vi "Feeder_Determiner.vi"() -> ()   [LabVIEW 2020]
uses:
  <vilib>/Rock Robotics/WPI/DriverStation/WPI_DriverStationRobotMode2.ctl
  Feeder_Control_States.ctl
  Subsystems/Funnel/Funnel_Cluster.ctl
  Subsystems/Funnel/Control_States_Funnel.ctl
  Subsystems/Magazine/Magazine_Cluster.ctl
  Subsystems/Magazine/Magazine_Control_States.ctl
  Subsystems/Intake/Intake_cluster.ctl
  Subsystems/Intake/Intake_control_states.ctl
  Globals/Feeder_Globals.vi
  Globals/Funnel_global.vi
  Globals/Magazine_Globals.vi
  Globals/Intake_Globals.vi
  Robot Global Data.vi
  Globals/Sensor_Values.vi
  Globals/Flywheel_Globals.vi
  Globals/Cowl_Globals.vi
  Shooter/Determiner/Shooter_Globals.vi
  Globals/Turret_Globals.vi
panel:
  in  "Intake_Outtake_%Vbus":dbl=-0.5
  in  "Magazine_Outtake_%Vbus":dbl=-0.3
  in  "Funnel_Outtake_%Vbus":dbl=-0.5
  in  "use magazine speed control test":bool
  in  "Magazine_Speed_Control_Test_Value":dbl=6000.0
  in  "Intake_Load_%Vbus":dbl=0.5
  in  "Magazine_Load_%Vbus":dbl=0.3
  in  "Funnel_Load_%Vbus":dbl=0.7
  in  "Funnel_Firing_%Vbus":dbl=0.5
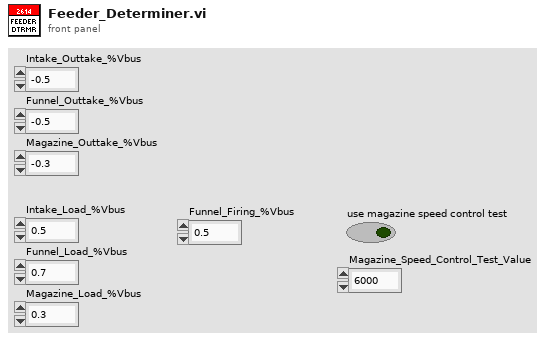
[diagram p1: front panel]
types:
  T1 = typedef "Feeder_Control_States.ctl" = enum16{"No-Op", "Manual", "Load", "Outtake", "Firing", "Test", "Command_Feed", "Command_Shoot", "Puke-Op", "Command_Feed_From_Pose", "Load+Firing", "Command_Puke"}
  T2 = typedef "Intake_cluster.ctl" = cluster{"control_states":T3, "%Vbus":dbl, "Trigger?":bool, "Manual_Extend?":bool, "Auto_Notifier":refnum<notifier>, "Step":dbl, "Parameter 1":dbl, "Parameter 2":dbl, "Parameter 3":dbl}
  T3 = typedef "Intake_control_states.ctl" = enum16{"No_Op", "Intake", "Manual", "Outtake", "Extend_No_Motor", "Retract_No_Motor"}
  T4 = typedef "Magazine_Cluster.ctl" = cluster{"Control_States":T5, "%Vbus":dbl, "Load_Magazine":bool, "Firing_Magazine":bool, "Velocity":dbl}
  T5 = typedef "Magazine_Control_States.ctl" = enum16{"No-Op", "Manual_%Vbus", "Manual_Speed_Control", "Test_Speed_Control", "Load", "Firing", "Outtake"}
  T6 = typedef "Funnel_Cluster.ctl" = cluster{"Control States":T7, "%Vbus":dbl}
  T7 = typedef "Control_States_Funnel.ctl" = enum16{"No_Op", "Manual_Op", "Load", "Firing", "Outtake"}
  T8 = typedef "WPI_DriverStationRobotMode2.ctl" = enum16{"Autonomous Disabled", "Autonomous Enabled", "Teleop Disabled", "Teleop Enabled", "Disconnected", "Finish", "Test Disabled", "Test Enabled", "Emergency Stopped"}
  T9 = typedef "Feeder_Cluster.ctl" = cluster{"Firing":bool, "Load":bool, "Magazine_%Vbus":dbl, "Funnel_%Vbus":dbl, "Intake_%Vbus":dbl, "Manual_Extend":bool, "Outtake":bool, "Parameters":dbl[], "Auto_Notifier":refnum<notifier>, "Step":i32, "Control_States":T1, "Puke?":bool}
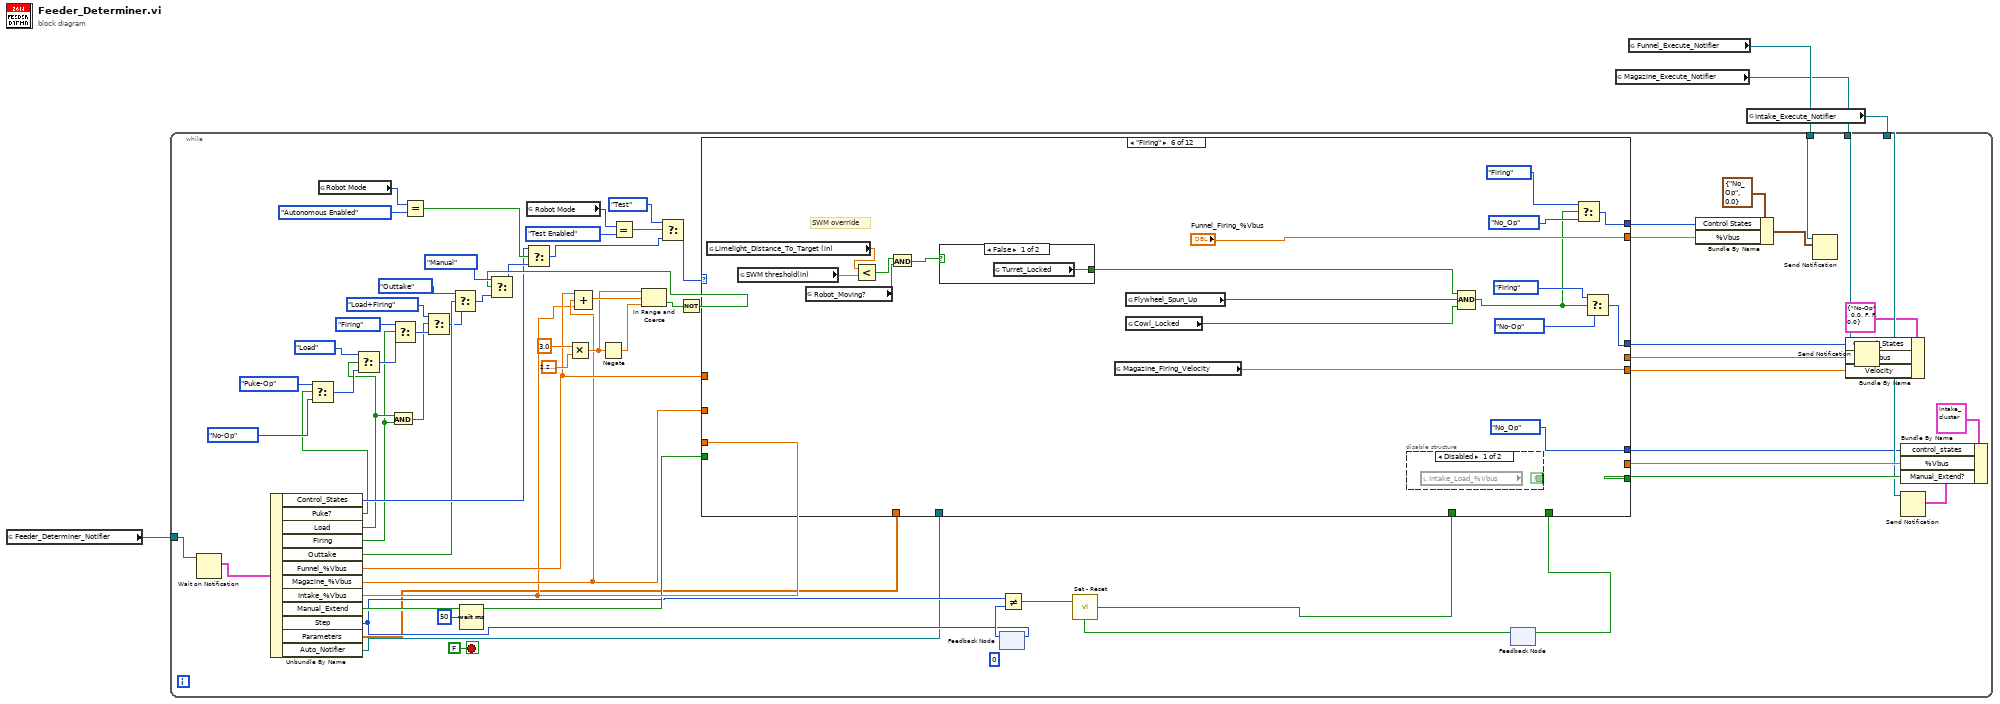
[diagram p0: block diagram]
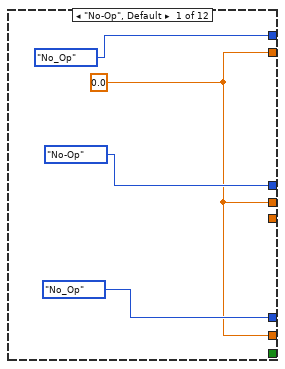
[diagram p2: hidden frame]
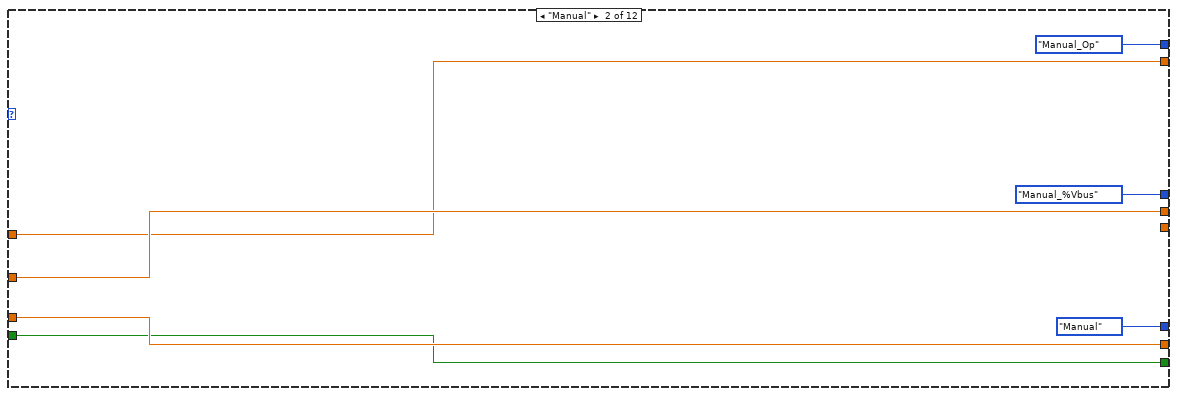
[diagram p3: hidden frame]
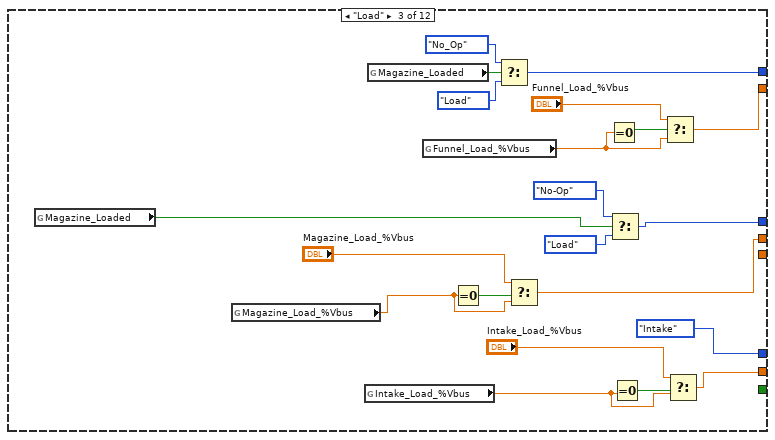
[diagram p4: hidden frame]
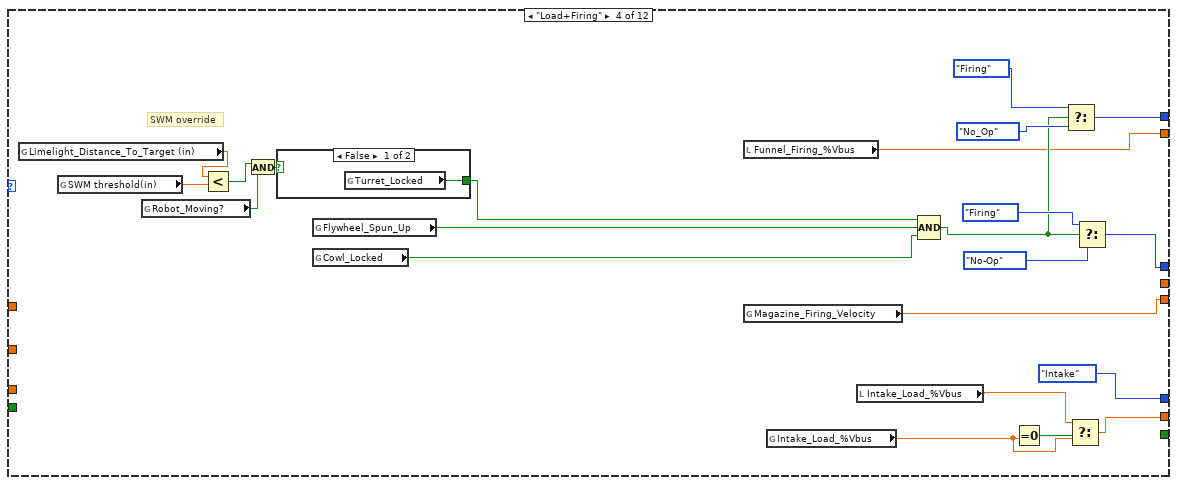
[diagram p5: hidden frame]
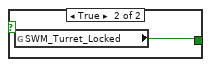
[diagram p6: hidden frame]
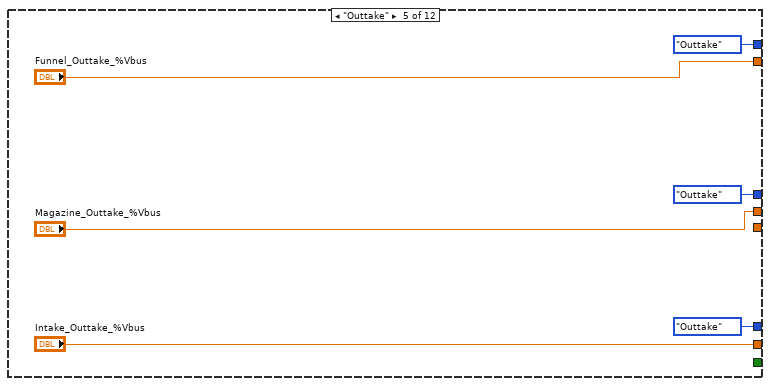
[diagram p7: hidden frame]
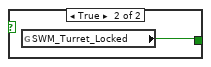
[diagram p8: hidden frame]
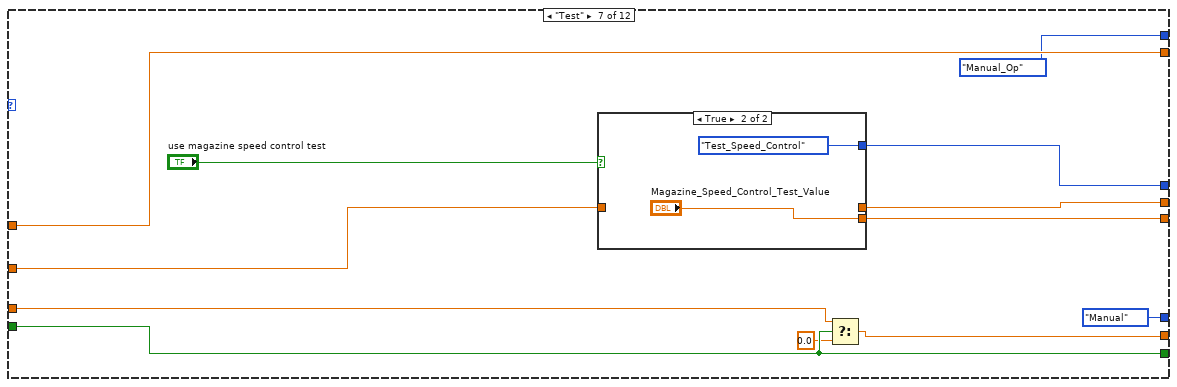
[diagram p10: hidden frame]
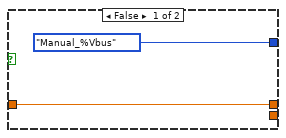
[diagram p11: hidden frame]
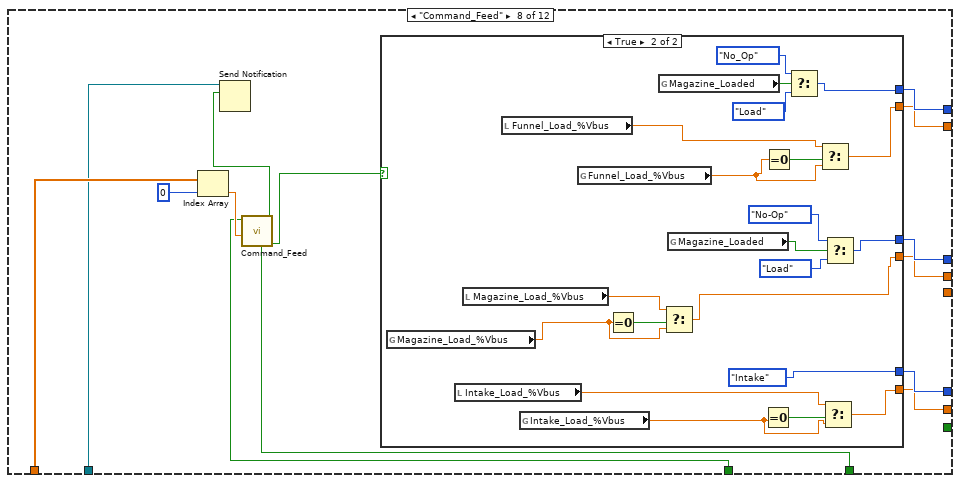
[diagram p12: hidden frame]
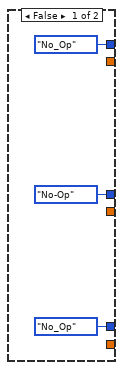
[diagram p13: hidden frame]
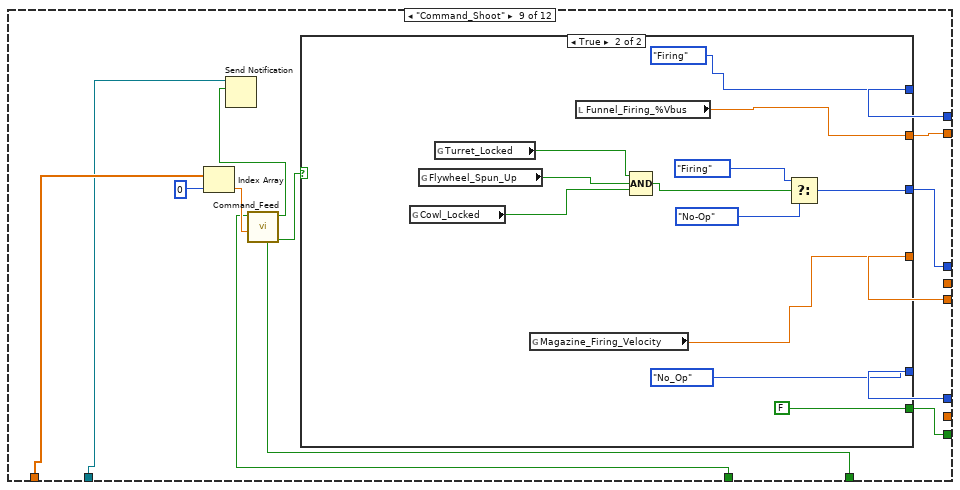
[diagram p14: hidden frame]
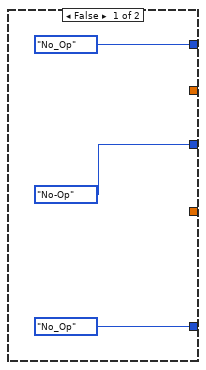
[diagram p15: hidden frame]
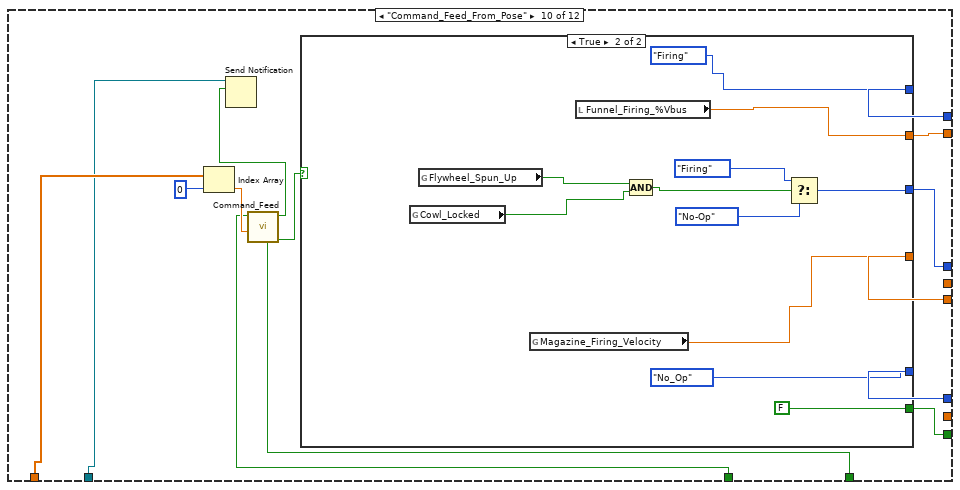
[diagram p16: hidden frame]
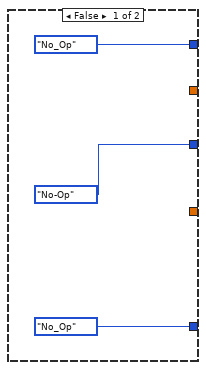
[diagram p17: hidden frame]
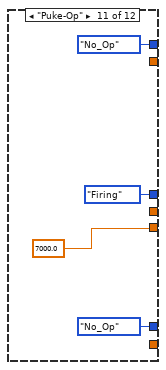
[diagram p18: hidden frame]
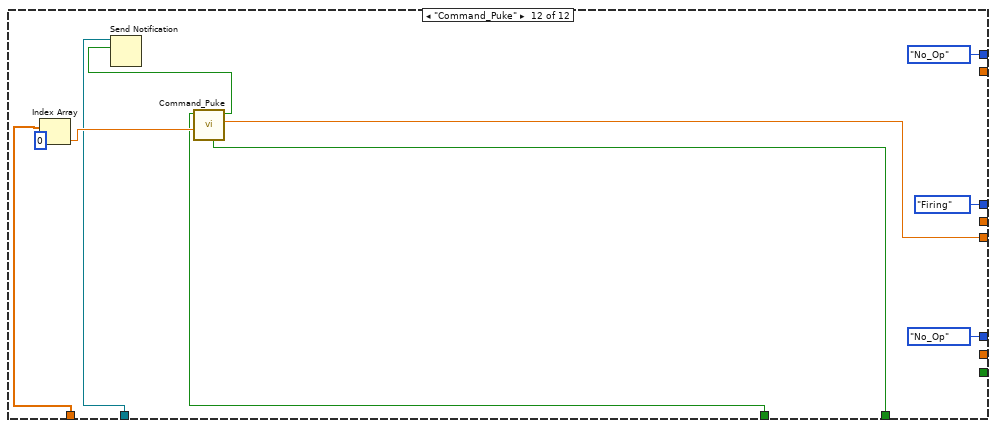
[diagram p19: hidden frame]
diagram:
  n1 = global read "Feeder_Globals.vi" "Feeder_Determiner_Notifier"() -> (w4:refnum<notifier>)
  n2 = global read "Magazine_Globals.vi" "Magazine_Execute_Notifier"() -> (w2:refnum<notifier>)
  n3 = global read "Funnel_global.vi" "Funnel_Execute_Notifier"() -> (w3:refnum<notifier>)
  n4 = global read "Intake_Globals.vi" "Intake_Execute_Notifier"() -> (w1:refnum<notifier>)
  n5 = while {
    tunnel: w4 -> [w71]
    tunnel: w3 -> [w59]
    tunnel: w2 -> [w58]
    tunnel: w1 -> [w57]
    stop <- FALSE stop-if-true
    (unwired) 0 ("Step")
    n6 = Wait on Notification(notifier=w71) -> (notification=w15:T9)  [unwired: 3 in, 3 out]
    n7 = Unbundle By Name(w15) -> ("Control_States"=w24:T1, "Puke?"=w9:bool, "Load"=w11:bool, "Firing"=w10:bool, "Outtake"=w23:bool, "Funnel_%Vbus"=w22:dbl, "Magazine_%Vbus"=w21:dbl, "Intake_%Vbus"=w20:dbl, "Manual_Extend"=w19:bool, "Step"=w18:i32, "Parameters"=w17:dbl[], "Auto_Notifier"=w16:refnum<notifier>)
    n8 = Select(t=Feeder_Control_States."Puke-Op", s=w9, f=Feeder_Control_States."No-Op" ("Control_States")) -> (s? t:f=w14:T1)
    n9 = global read "Robot Global Data.vi" "Robot Mode"() -> (w46:T8)
    n10 = Select(t=Feeder_Control_States."Load" ("Control_States"), s=w11, f=w14) -> (s? t:f=w67:T1)
    n11 = And(x=w11, y=w10) -> (x .and. y?=w7:bool)
    n12 = Select(t=Feeder_Control_States."Firing" ("Control_States"), s=w10, f=w67) -> (s? t:f=w8:T1)
    n13 = Equal?(x=w46, y=WPI_DriverStationRobotMode2."Autonomous Enabled" ("Robot Mode")) -> (x = y?=w35:bool)
    n14 = Select(t=Feeder_Control_States."Load+Firing" ("Control_States"), s=w7, f=w8) -> (s? t:f=w5:T1)
    n15 = Select(t=Feeder_Control_States."Outtake" ("Control_States"), s=w23, f=w5) -> (s? t:f=w34:T1)
    n16 = Wait (ms)(milliseconds to wait=u32 50) -> ()  [unwired: 1 out]
    n17 = global read "Robot Global Data.vi" "Robot Mode"() -> (w69:T8)
    n18 = Multiply(x=3.0, y=2.220446049250313e-16) -> (x*y=w28:dbl)
    n19 = Compound Arithmetic op=ADD(w22, w21, w20) -> (w32:dbl)
    n20 = Negate(x=w28) -> (-x=w31:dbl)
    n21 = Equal?(x=w69, y=WPI_DriverStationRobotMode2."Test Enabled" ("Robot Mode")) -> (x = y?=w68:bool)
    n22 = In Range and Coerce(upper limit=w28, x=w32, lower limit=w31) -> (In Range?=w27:bool)  [unwired: 1 out]
    n23 = Not(x=w27) -> (.not. x?=w26:bool)
    n24 = Select(t=Feeder_Control_States."Manual", s=w26, f=w34) -> (s? t:f=w25:T1)
    n25 = Select(t=w24, s=w35, f=w25) -> (s? t:f=w45:T1)
    n26 = Select(t=Feeder_Control_States."Test" ("Control_States"), s=w68, f=w45) -> (s? t:f=w60:T1)
    n27 = feedback #1() -> (w42:i32)  [unwired: 1 in]
    n28 = feedback-in #1(w18) -> ()
    n29 = Not Equal?(x=w18, y=w42) -> (x != y?=w43:bool)
    n30 = feedback #2() -> (w44:bool)  [unwired: 1 in]
    n31 = call "Set - Reset.vi"("Reset"=w44, "Set"=w43) -> ("Output"=w40:bool)
    n32 = case shown="\"Firing\"" w60 {
      tunnel: [Magazine_Control_States."No-Op" ("Control_States") Magazine_Control_States."Manual_%Vbus" ("Control_States") w97 w112 Magazine_Control_States."Outtake" ("Control_States") w149 w167 w176 w214 w243 Magazine_Control_States."Firing" ("Control_States") Magazine_Control_States."Firing" ("Control_States")] -> w64
      tunnel: [Intake_control_states."No_Op" ("control_states") Intake_control_states."Manual" ("control_states") Intake_control_states."Intake" ("control_states") Intake_control_states."Intake" ("control_states") Intake_control_states."Outtake" ("control_states") Intake_control_states."No_Op" ("control_states") Intake_control_states."Manual" ("control_states") w175 w211 w240 Intake_control_states."No_Op" ("control_states") Intake_control_states."No_Op" ("control_states")] -> w37
      tunnel: [w74 w82 w84 w123 "Intake_Outtake_%Vbus" _ w157 w172 _ _ _ _] -> w62
      tunnel: [_ w81 _ _ _ _ w159 _ w215 w244 _ _] -> w61
      tunnel: w22 -> [_ w79 _ _ _ _ w166 _ _ _ _ _]
      tunnel: [w74 w79 w92 w114 "Funnel_Outtake_%Vbus" "Funnel_Firing_%Vbus" w166 w174 w210 w239 _ _] -> w56
      tunnel: w21 -> [_ w83 _ _ _ _ w165 _ _ _ _ _]
      tunnel: [w74 w83 w88 _ "Magazine_Outtake_%Vbus" _ w163 w173 _ _ _ _] -> w55
      tunnel: w20 -> [_ w82 _ _ _ _ w158 _ _ _ _ _]
      tunnel: w19 -> [_ w81 _ _ _ _ w159 _ _ _ _ _]
      tunnel: [_ _ _ w111 _ w141 w162 _ w213 w242 7000.0 ("Magazine_Firing_Velocity") w271] -> w53
      tunnel: [Control_States_Funnel."No_Op" ("Control States") Control_States_Funnel."Manual_Op" ("Control States") w96 w113 Control_States_Funnel."Outtake" ("Control States") w145 Control_States_Funnel."Manual_Op" ("Control States") w177 w212 w241 Control_States_Funnel."No_Op" ("Control States") Control_States_Funnel."No_Op" ("Control States")] -> w48
      tunnel: w17 -> [_ _ _ _ _ _ _ w185 w219 w248 _ w280]
      tunnel: w40 -> [_ _ _ _ _ _ _ w182 w216 w245 _ w278]
      tunnel: [_ _ _ _ _ _ _ w181 w217 w246 _ w277] -> w41
      tunnel: w16 -> [_ _ _ _ _ _ _ w180 w218 w247 _ w275]
      frame "No-Op", Default {
        w74 = 0.0 ("Throttle")
      }
      frame "Manual" {
      }
      frame "Load" {
        n33 = global read "Sensor_Values.vi" "Magazine_Loaded"() -> (w100:bool)
        n34 = global read "Feeder_Globals.vi" "Magazine_Load_%Vbus"() -> (w89:dbl)
        n35 = global read "Feeder_Globals.vi" "Intake_Load_%Vbus"() -> (w85:dbl)
        n36 = global read "Sensor_Values.vi" "Magazine_Loaded"() -> (w101:bool)
        n37 = global read "Feeder_Globals.vi" "Funnel_Load_%Vbus"() -> (w93:dbl)
        n38 = Equal To 0?(x=w89) -> (x = 0?=w90:bool)
        n39 = Select(t=Control_States_Funnel."No_Op" ("Control States"), s=w101, f=Control_States_Funnel."Load" ("Control States")) -> (s? t:f=w96:T7)
        n40 = Select(t="Magazine_Load_%Vbus", s=w90, f=w89) -> (s? t:f=w88:dbl)
        n41 = Equal To 0?(x=w93) -> (x = 0?=w95:bool)
        n42 = Select(t=Magazine_Control_States."No-Op" ("Control_States"), s=w100, f=Magazine_Control_States."Load" ("Control_States")) -> (s? t:f=w97:T5)
        n43 = Equal To 0?(x=w85) -> (x = 0?=w87:bool)
        n44 = Select(t="Funnel_Load_%Vbus", s=w95, f=w93) -> (s? t:f=w92:dbl)
        n45 = Select(t="Intake_Load_%Vbus", s=w87, f=w85) -> (s? t:f=w84:dbl)
      }
      frame "Load+Firing" {
        # "SWM override"
        n46 = global read "Sensor_Values.vi" "Limelight_Distance_To_Target (in)"() -> (w108:dbl)
        n47 = global read "Shooter_Globals.vi" "SWM threshold(in)"() -> (w107:dbl)
        n48 = global read "Sensor_Values.vi" "Robot_Moving?"() -> (w109:bool)
        n49 = Less?(x=w108, y=w107) -> (x < y?=w106:bool)
        n50 = And(x=w106, y=w109) -> (x .and. y?=w110:bool)
        n51 = case shown="False" w110 {
          tunnel: [w127 w128] -> w105
          frame False {
            n52 = global read "Turret_Globals.vi" "Turret_Locked"() -> (w127:bool)
          }
          frame True {
            n53 = global read "Turret_Globals.vi" "SWM_Turret_Locked"() -> (w128:bool)
          }
        }
        n54 = global read "Flywheel_Globals.vi" "Flywheel_Spun_Up"() -> (w117:bool)
        n55 = global read "Cowl_Globals.vi" "Cowl_Locked"() -> (w115:bool)
        n56 = local read "Funnel_Firing_%Vbus"() -> (w114:dbl)
        n57 = global read "Feeder_Globals.vi" "Magazine_Firing_Velocity"() -> (w111:dbl)
        n58 = global read "Feeder_Globals.vi" "Intake_Load_%Vbus"() -> (w124:dbl)
        n59 = local read "Intake_Load_%Vbus"() -> (w122:dbl)
        n60 = Compound Arithmetic op=AND(w105, w117, w115) -> (w116:bool)
        n61 = Equal To 0?(x=w124) -> (x = 0?=w125:bool)
        n62 = Select(t=Control_States_Funnel."Firing" ("Control States"), s=w116, f=Control_States_Funnel."No_Op" ("Control States")) -> (s? t:f=w113:T7)
        n63 = Select(t=w122, s=w125, f=w124) -> (s? t:f=w123:dbl)
        n64 = Select(t=Magazine_Control_States."Firing" ("Control_States"), s=w116, f=Magazine_Control_States."No-Op" ("Control_States")) -> (s? t:f=w112:T5)
      }
      frame "Outtake" {
      }
      frame "Firing" {
        # "SWM override"
        n65 = global read "Sensor_Values.vi" "Limelight_Distance_To_Target (in)"() -> (w137:dbl)
        n66 = global read "Shooter_Globals.vi" "SWM threshold(in)"() -> (w136:dbl)
        n67 = global read "Sensor_Values.vi" "Robot_Moving?"() -> (w138:bool)
        n68 = Less?(x=w137, y=w136) -> (x < y?=w135:bool)
        n69 = And(x=w135, y=w138) -> (x .and. y?=w139:bool)
        n70 = case shown="False" w139 {
          tunnel: [w153 w154] -> w140
          frame False {
            n71 = global read "Turret_Globals.vi" "Turret_Locked"() -> (w153:bool)
          }
          frame True {
            n72 = global read "Turret_Globals.vi" "SWM_Turret_Locked"() -> (w154:bool)
          }
        }
        n73 = global read "Feeder_Globals.vi" "Magazine_Firing_Velocity"() -> (w141:dbl)
        n74 = global read "Flywheel_Globals.vi" "Flywheel_Spun_Up"() -> (w144:bool)
        n75 = global read "Cowl_Globals.vi" "Cowl_Locked"() -> (w142:bool)
        n76 = disable-structure shown="Disabled" {
          disable-tunnel: [FALSE ("intake_extended") _] -> _
          frame Disabled {
            n77 = local read "Intake_Load_%Vbus"() -> ()  [unwired: 1 out]
          }
          frame Enabled {
          }
        }
        n78 = Compound Arithmetic op=AND(w140, w144, w142) -> (w143:bool)
        n79 = Select(t=Control_States_Funnel."Firing" ("Control States"), s=w143, f=Control_States_Funnel."No_Op" ("Control States")) -> (s? t:f=w145:T7)
        n80 = Select(t=Magazine_Control_States."Firing" ("Control_States"), s=w143, f=Magazine_Control_States."No-Op" ("Control_States")) -> (s? t:f=w149:T5)
      }
      frame "Test" {
        n81 = case shown="True" "use magazine speed control test" {
          tunnel: [Magazine_Control_States."Manual_%Vbus" ("Control_States") Magazine_Control_States."Test_Speed_Control" ("Control_States")] -> w167
          tunnel: [w168 _] -> w163
          tunnel: w165 -> [w168 _]
          tunnel: [_ "Magazine_Speed_Control_Test_Value"] -> w162
          frame False {
          }
          frame True {
          }
        }
        n82 = Select(t=w158, s=w159, f=0.0) -> (s? t:f=w157:dbl)
      }
      frame "Command_Feed" {
        n83 = Index Array(array=w185, index=0) -> (element=w183:dbl)
        n84 = call "Command_Feed.vi"("Startup"=w182, "Timeout"=w183) -> ("Reint"=w181:bool, "Completed"=w179:bool, "Output"=w178:bool)  [unwired: 6 in]
        n85 = Send Notification(notification=w179, notifier=w180) -> ()  [unwired: 1 in, 2 out]
        n86 = case shown="True" w178 {
          tunnel: [Control_States_Funnel."No_Op" ("Control States") w203] -> w177
          tunnel: [Magazine_Control_States."No-Op" ("Control_States") w202] -> w176
          tunnel: [Intake_control_states."No_Op" ("control_states") Intake_control_states."Intake" ("control_states")] -> w175
          tunnel: [_ w189] -> w174
          tunnel: [_ w193] -> w173
          tunnel: [_ w197] -> w172
          frame False {
          }
          frame True {
            n87 = global read "Feeder_Globals.vi" "Magazine_Load_%Vbus"() -> (w194:dbl)
            n88 = local read "Intake_Load_%Vbus"() -> (w199:dbl)
            n89 = local read "Magazine_Load_%Vbus"() -> (w195:dbl)
            n90 = local read "Funnel_Load_%Vbus"() -> (w191:dbl)
            n91 = global read "Feeder_Globals.vi" "Intake_Load_%Vbus"() -> (w198:dbl)
            n92 = global read "Feeder_Globals.vi" "Funnel_Load_%Vbus"() -> (w190:dbl)
            n93 = Equal To 0?(x=w194) -> (x = 0?=w196:bool)
            n94 = global read "Sensor_Values.vi" "Magazine_Loaded"() -> (w207:bool)
            n95 = Select(t=w195, s=w196, f=w194) -> (s? t:f=w193:dbl)
            n96 = global read "Sensor_Values.vi" "Magazine_Loaded"() -> (w206:bool)
            n97 = Equal To 0?(x=w198) -> (x = 0?=w200:bool)
            n98 = Equal To 0?(x=w190) -> (x = 0?=w192:bool)
            n99 = Select(t=Control_States_Funnel."No_Op" ("Control States"), s=w207, f=Control_States_Funnel."Load" ("Control States")) -> (s? t:f=w203:T7)
            n100 = Select(t=w191, s=w192, f=w190) -> (s? t:f=w189:dbl)
            n101 = Select(t=w199, s=w200, f=w198) -> (s? t:f=w197:dbl)
            n102 = Select(t=Magazine_Control_States."No-Op" ("Control_States"), s=w206, f=Magazine_Control_States."Load" ("Control_States")) -> (s? t:f=w202:T5)
          }
        }
      }
      frame "Command_Shoot" {
        n103 = Index Array(array=w219, index=0) -> (element=w222:dbl)
        n104 = call "Command_Feed.vi"("Startup"=w216, "Timeout"=w222) -> ("Reint"=w217:bool, "Completed"=w221:bool, "Output"=w220:bool)  [unwired: 6 in]
        n105 = Send Notification(notification=w221, notifier=w218) -> ()  [unwired: 1 in, 2 out]
        n106 = case shown="True" w220 {
          tunnel: [Control_States_Funnel."No_Op" ("Control States") Control_States_Funnel."Firing" ("Control States")] -> w212
          tunnel: [Intake_control_states."No_Op" ("control_states") Intake_control_states."No_Op" ("control_states")] -> w211
          tunnel: [_ w227] -> w213
          tunnel: [_ FALSE] -> w215
          tunnel: [Magazine_Control_States."No-Op" ("Control_States") w231] -> w214
          tunnel: [_ w236] -> w210
          frame False {
          }
          frame True {
            n107 = global read "Cowl_Globals.vi" "Cowl_Locked"() -> (w228:bool)
            n108 = global read "Flywheel_Globals.vi" "Flywheel_Spun_Up"() -> (w233:bool)
            n109 = global read "Turret_Globals.vi" "Turret_Locked"() -> (w229:bool)
            n110 = global read "Feeder_Globals.vi" "Magazine_Firing_Velocity"() -> (w227:dbl)
            n111 = local read "Funnel_Firing_%Vbus"() -> (w236:dbl)
            n112 = Compound Arithmetic op=AND(w229, w233, w228) -> (w232:bool)
            n113 = Select(t=Magazine_Control_States."Firing" ("Control_States"), s=w232, f=Magazine_Control_States."No-Op" ("Control_States")) -> (s? t:f=w231:T5)
          }
        }
      }
      frame "Command_Feed_From_Pose" {
        n114 = Index Array(array=w248, index=0) -> (element=w251:dbl)
        n115 = call "Command_Feed.vi"("Startup"=w245, "Timeout"=w251) -> ("Reint"=w246:bool, "Completed"=w250:bool, "Output"=w249:bool)  [unwired: 6 in]
        n116 = Send Notification(notification=w250, notifier=w247) -> ()  [unwired: 1 in, 2 out]
        n117 = case shown="True" w249 {
          tunnel: [Control_States_Funnel."No_Op" ("Control States") Control_States_Funnel."Firing" ("Control States")] -> w241
          tunnel: [Intake_control_states."No_Op" ("control_states") Intake_control_states."No_Op" ("control_states")] -> w240
          tunnel: [_ w258] -> w242
          tunnel: [_ FALSE] -> w244
          tunnel: [Magazine_Control_States."No-Op" ("Control_States") w260] -> w243
          tunnel: [_ w264] -> w239
          frame False {
          }
          frame True {
            n118 = global read "Cowl_Globals.vi" "Cowl_Locked"() -> (w256:bool)
            n119 = global read "Flywheel_Globals.vi" "Flywheel_Spun_Up"() -> (w257:bool)
            n120 = global read "Feeder_Globals.vi" "Magazine_Firing_Velocity"() -> (w258:dbl)
            n121 = local read "Funnel_Firing_%Vbus"() -> (w264:dbl)
            n122 = Compound Arithmetic op=AND(w257, w256) -> (w261:bool)
            n123 = Select(t=Magazine_Control_States."Firing" ("Control_States"), s=w261, f=Magazine_Control_States."No-Op" ("Control_States")) -> (s? t:f=w260:T5)
          }
        }
      }
      frame "Puke-Op" {
      }
      frame "Command_Puke" {
        n124 = Index Array(array=w280, index=0) -> (element=w279:dbl)
        n125 = call "Command_Puke.vi"("Startup"=w278, "Timeout"=w279) -> ("Reint"=w277:bool, "Completed"=w276:bool, "Magazine_Velocity"=w271:dbl)  [unwired: 6 in]
        n126 = Send Notification(notification=w276, notifier=w275) -> ()  [unwired: 1 in, 2 out]
      }
    }
    n127 = feedback-in #2(w41) -> ()
    n128 = Bundle By Name(cluster=T6 {"Control States"=enum."No_Op", "%Vbus"=0.0} ("Funnel_Cluster"), "Control States"=w48, "%Vbus"=w56) -> (w66:T6)
    n129 = Send Notification(notification=w66, notifier=w59) -> ()  [unwired: 1 in, 2 out]
    n130 = Bundle By Name(cluster=T4 {"Control_States"=enum."No-Op", "%Vbus"=0.0, "Load_Magazine"=FALSE, "Firing_Magazine"=FALSE, "Velocity"=0.0} ("Magazine_Cluster"), "Control_States"=w64, "%Vbus"=w55, "Velocity"=w53) -> (w65:T4)
    n131 = Send Notification(notification=w65, notifier=w58) -> ()  [unwired: 1 in, 2 out]
    n132 = Bundle By Name(cluster=T2 {"control_states"=enum."No_Op", "%Vbus"=0.0, "Trigger?"=FALSE, "Manual_Extend?"=FALSE, "Auto_Notifier"=refnum, "Step"=0.0, "Parameter 1"=0.0, "Parameter 2"=0.0, "Parameter 3"=0.0} ("Intake_cluster"), "control_states"=w37, "%Vbus"=w62, "Manual_Extend?"=w61) -> (w63:T2)
    n133 = Send Notification(notification=w63, notifier=w57) -> ()  [unwired: 1 in, 2 out]
  }
